vi "Wait Event Callback.vi"(4 "Main VI Refnum":refnum<vi>, 5 "Event data":cluster{"showWait":bool}, 6 "CtlRef":refnum<k7>, 7 "Event common data":cluster{"Source":i32, "Type":u32, "Time":u32}) -> ()   [LabVIEW 2010, in "TS Simple LabVIEW OI Dependencies.lvlib"]
uses:
  TS Simple LabVIEW OI Dependencies.lvlib
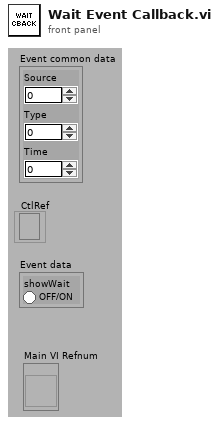
[diagram p1: front panel]
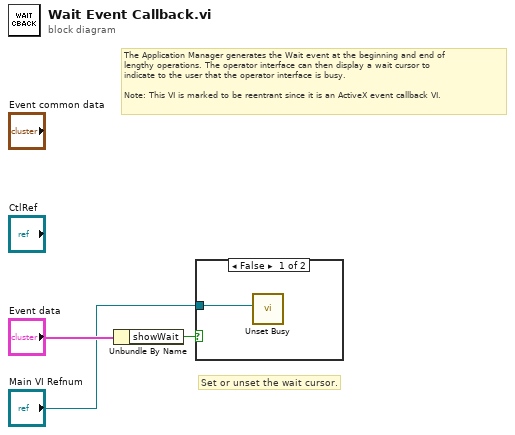
[diagram p0: block diagram]
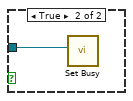
[diagram p2: hidden frame]
diagram:
  # "Set or unset the wait cursor."
  # "The Application Manager generates the Wait event at the beginning and end of\nlengthy operations. The operator interface can then display a wait cursor to\nindicate to the user that the operator interface is busy.\n\nNote: This VI is marked to be reentrant since it is an ActiveX event callback VI."
  n1 = Unbundle By Name("Event data") -> ("showWait"=w3:bool)
  n2 = case shown="False" w3 {
    tunnel: "Main VI Refnum" -> [w4 w5]
    frame False {
      n3 = call <vilib>:"Unset Busy.vi"("VI reference (current VI)"=w4) -> ()  [unwired: 1 in, 10 out]
    }
    frame True {
      n4 = call <vilib>:"Set Busy.vi"("VI reference (current VI)"=w5) -> ()  [unwired: 3 in, 8 out]
    }
  }
